vi "Main.vi"() -> ()   [LabVIEW 2017]
uses:
  CTL/REF Channel Select.ctl
  D:/test/ILSTS/LV_IL_Sample/DLL/STSProcess.dll
  DLL/STSProcess.dll
  CTL/Address Cluster.ctl
  D:/test/ILSTS/LV_IL_Sample/DLL/InstrumentDLL.dll
  DLL/InstrumentDLL.dll
  <vilib>/Utility/miscctls.llb/LVStringsAndValuesArrayTypeDef_DBL.ctl
panel:
  in  "ILSTS":refnum<k24>
  in  "btnzeroing":bool
  in  "btnreadref_data":bool
  in  "btnsaveRawdata":bool
  in  "btnsaveref_rawdata":bool
  in  "chkeach_ch":bool
  in  "btnmeas":bool
  in  "btnset":bool
  in  "Range1":bool
  in  "REF Channel Select":T1={"M1S0C1"=TRUE, "M1S0C2"=FALSE, "M1S0C3"=FALSE, "M1S0C4"=FALSE, "M1S1C1"=FALSE, "M1S1C2"=FALSE, "M1S1C3"=FALSE, "M1S1C4"=FALSE, "M1S2C1"=FALSE, "M1S2C2"=FALSE, "M1S2C3"=FALSE, "M1S2C4"=FALSE, "M1S3C1"=FALSE, "M1S3C2"=FALSE, "M1S3C3"=FALSE, "M1S3C4"=FALSE, "M1S4C1"=FALSE, "M1S4C2"=FALSE, "M1S4C3"=FALSE, "M1S4C4"=FALSE, "M2S0C1"=FALSE, "M2S0C2"=FALSE, "M2S0C3"=FALSE, "M2S0C4"=FALSE, "M2S1C1"=FALSE, "M2S1C2"=FALSE, "M2S1C3"=FALSE, "M2S1C4"=FALSE, "M2S2C1"=FALSE, "M2S2C2"=FALSE, "M2S2C3"=FALSE, "M2S2C4"=FALSE, "M2S3C1"=FALSE, "M2S3C2"=FALSE, "M2S3C3"=FALSE, "M2S3C4"=FALSE, "M2S4C1"=FALSE, "M2S4C2"=FALSE, "M2S4C3"=FALSE, "M2S4C4"=FALSE}
  in  "Range2":bool
  in  "Range3":bool
  in  "Range4":bool
  in  "Range5":bool
  in  "btnget_reference":bool
  in  "Address Cluster":T2={"SPU"=refnum, "MPM"=[], "Port_Count"=0.0, "MPM_Count"=0.0, "SPU_Resource"=[], "USB_Resource"=[], "MPM_Communicater"="", "MPM_Count"=0.0, "MPM_Address"=[], "MPM_Portnumber"=[], "SPU_DeviveID"="", "MPM_communcation_method"=[], "TSL_sweepstartwave"=0.0, "TSL_sweepstopwave"=0.0, "TSL_Address"="", "TSL_Communicater"="", "TSL"=refnum, "tsl_communcation_method"=3, "TSL_Portnumber"=0.0} {"tsl_communcation_method" items=["GPIB", "C232C", "TCPIP", "USB"]; "MPM_communcation_method" items=["GPIB", "C232C", "TCPIP", "USB"]}
  in  "Active Sensors":bool[](array[boolean])
  out "Meas_rang":i32[](array[numeric])
  out "Flag_213":bool
  out "Flag_215":bool
  out "Mergedata_struct":refnum<k24>[](array[refnum])
  out "Meas_monitor_struct":refnum<k24>[](array[refnum])
  out "Ref_monitordata_struct":refnum<k24>[](array[refnum])
  out "Refdata_struct":refnum<k24>[](array[refnum])
  out "Data_struct":refnum<k24>[](array[refnum])
  in  "txtpower":dbl caption="TSL Power(dBm)"
  in  "cmbspeed":u16(ring) caption="SweepSpeed(nm/sec)" items=["1"=1, "5"=5, "10"=10, "20"=20, "40"=40, "50"=50, "80"=80, "100"=100]
  in  "txtstepwave":dbl caption="WavelengthStep(nm)"
  in  "txtstopwave":dbl caption="StopWavelength(nm)"
  in  "txtstartwave":dbl caption="StartWavelength(nm)"
  # "Measurement ch"
  # "Measurement Range"
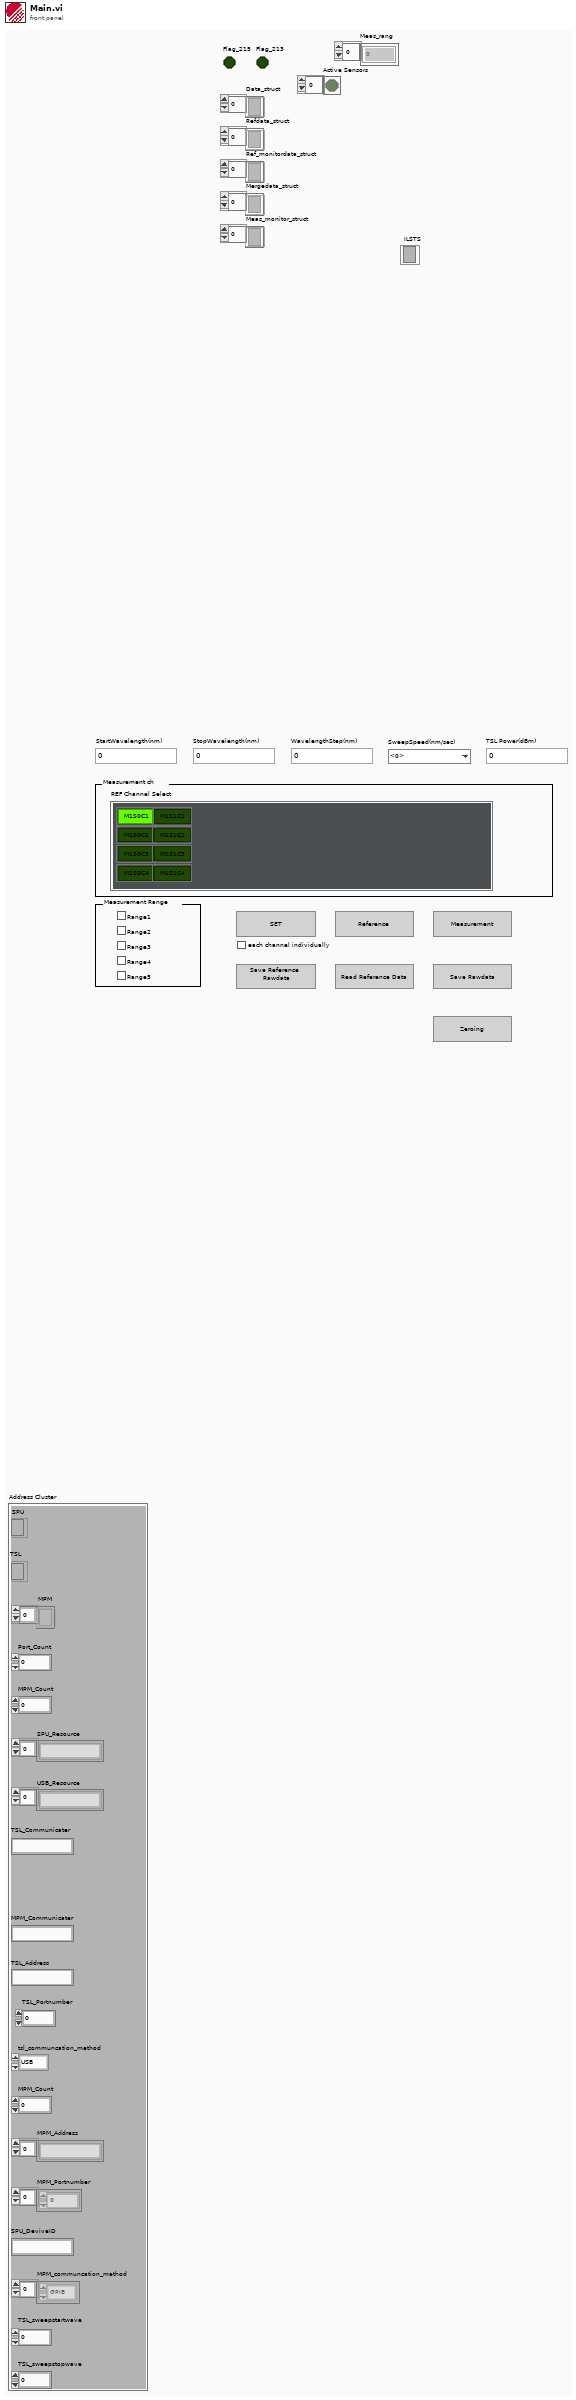
[diagram p1: front panel]
types:
  T1 = typedef "REF Channel Select.ctl" = cluster{"M1S0C1":bool, "M1S0C2":bool, "M1S0C3":bool, "M1S0C4":bool, "M1S1C1":bool, "M1S1C2":bool, "M1S1C3":bool, "M1S1C4":bool, "M1S2C1":bool, "M1S2C2":bool, "M1S2C3":bool, "M1S2C4":bool, "M1S3C1":bool, "M1S3C2":bool, "M1S3C3":bool, "M1S3C4":bool, "M1S4C1":bool, "M1S4C2":bool, "M1S4C3":bool, "M1S4C4":bool, "M2S0C1":bool, "M2S0C2":bool, "M2S0C3":bool, "M2S0C4":bool, "M2S1C1":bool, "M2S1C2":bool, "M2S1C3":bool, "M2S1C4":bool, "M2S2C1":bool, "M2S2C2":bool, "M2S2C3":bool, "M2S2C4":bool, "M2S3C1":bool, "M2S3C2":bool, "M2S3C3":bool, "M2S3C4":bool, "M2S4C1":bool, "M2S4C2":bool, "M2S4C3":bool, "M2S4C4":bool}
  T2 = typedef "Address Cluster.ctl" = cluster{"SPU":refnum<k24>, "MPM":refnum<k24>[], "Port_Count":dbl, "MPM_Count":dbl, "SPU_Resource":string[], "USB_Resource":string[], "MPM_Communicater":string, "MPM_Count":dbl, "MPM_Address":string[], "MPM_Portnumber":dbl[], "SPU_DeviveID":string, "MPM_communcation_method":i32[], "TSL_sweepstartwave":dbl, "TSL_sweepstopwave":dbl, "TSL_Address":string, "TSL_Communicater":string, "TSL":refnum<k24>, "tsl_communcation_method":i32, "TSL_Portnumber":dbl}
  T3 = enum8{"Enabled", "Disabled", "Disabled and Grayed Out"}
  T4 = typedef "LVStringsAndValuesArrayTypeDef_DBL.ctl" = cluster{"String":string, "Value":dbl}[]
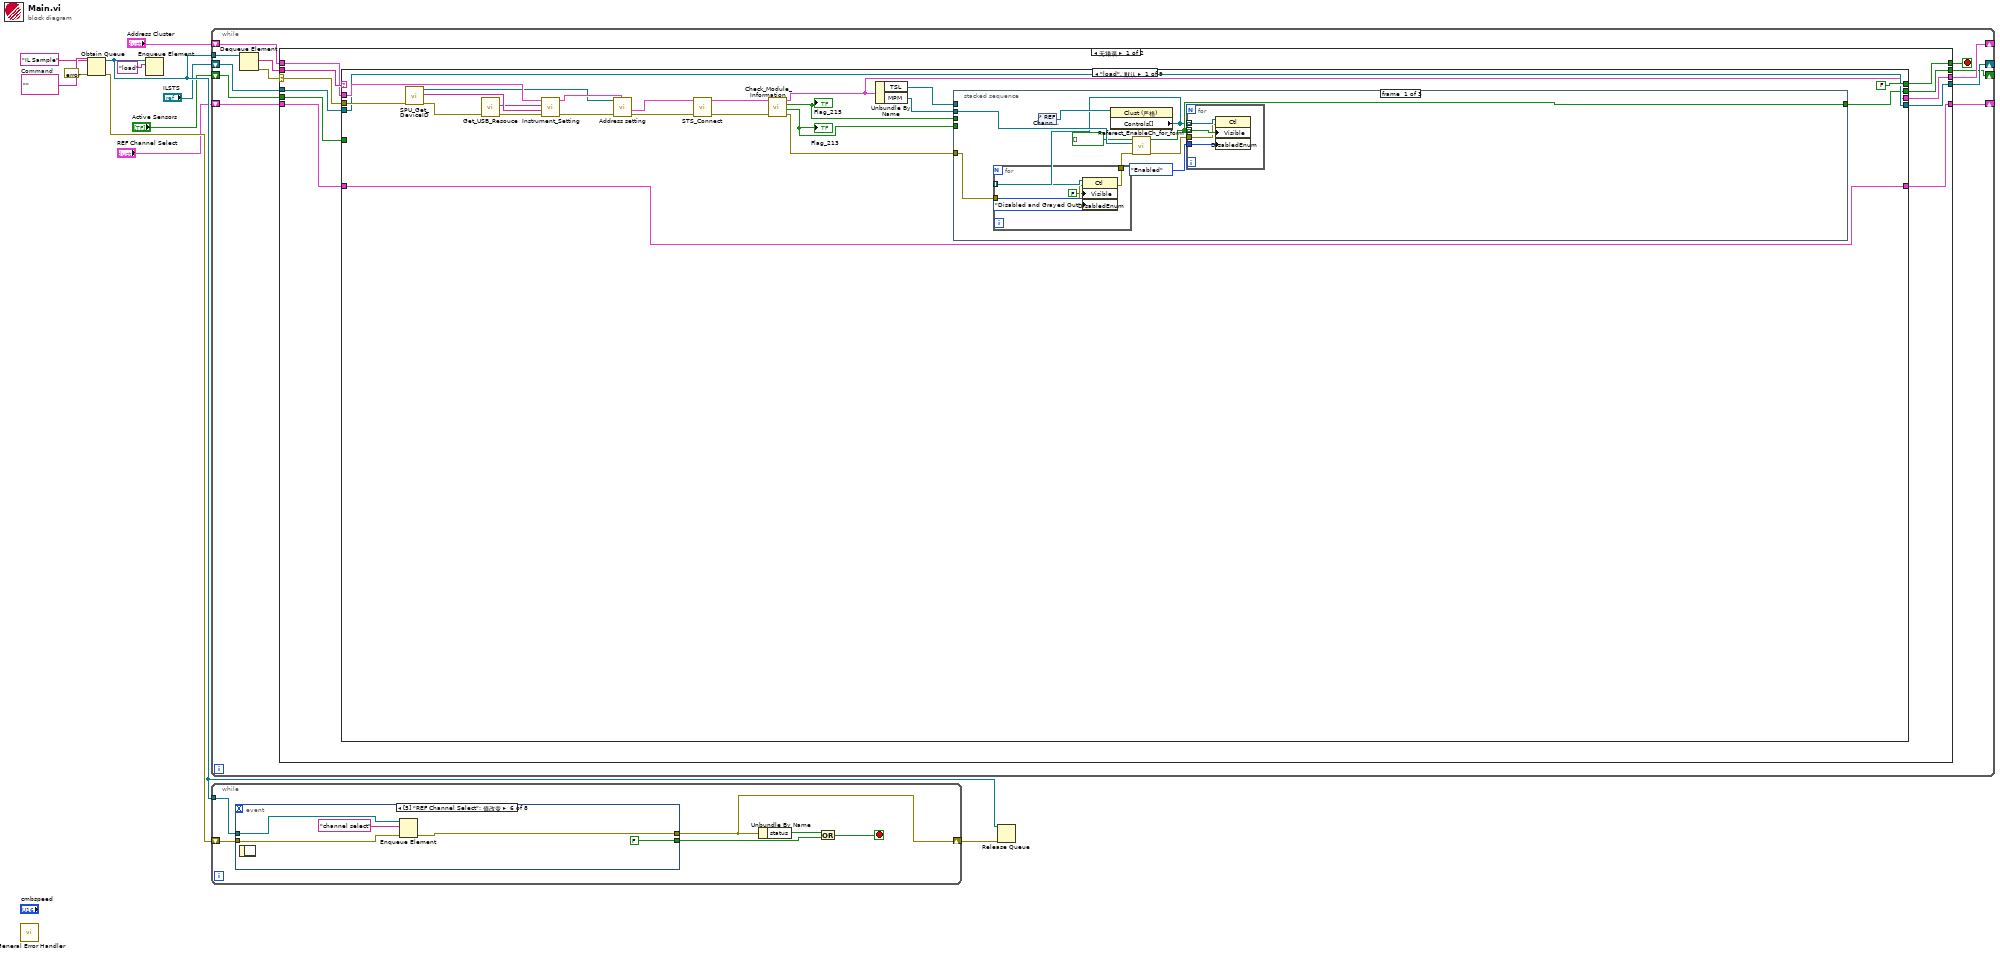
[diagram p0: block diagram]
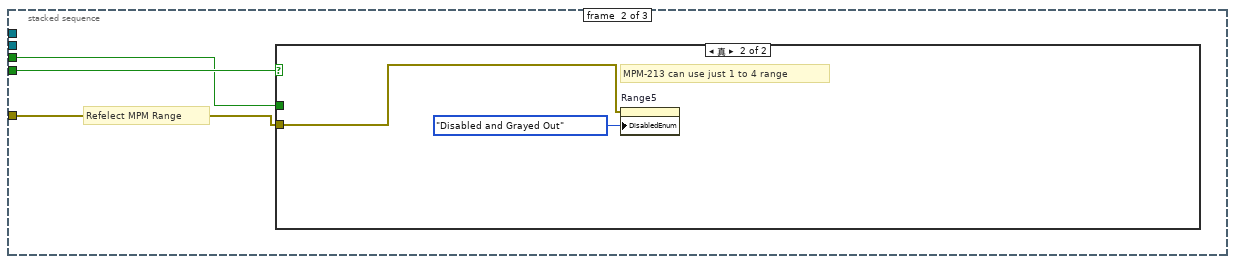
[diagram p2: hidden frame]
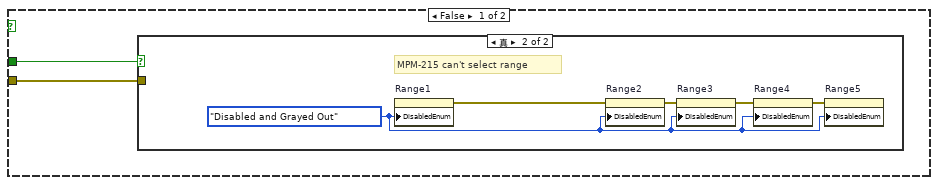
[diagram p3: hidden frame]
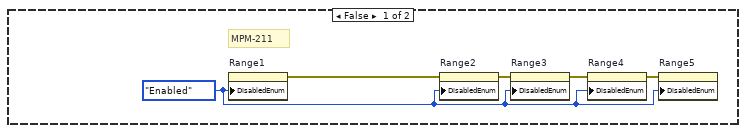
[diagram p4: hidden frame]
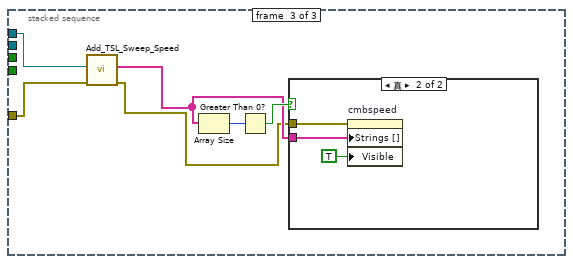
[diagram p5: hidden frame]
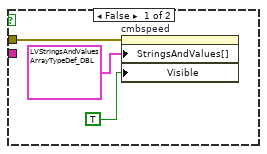
[diagram p6: hidden frame]
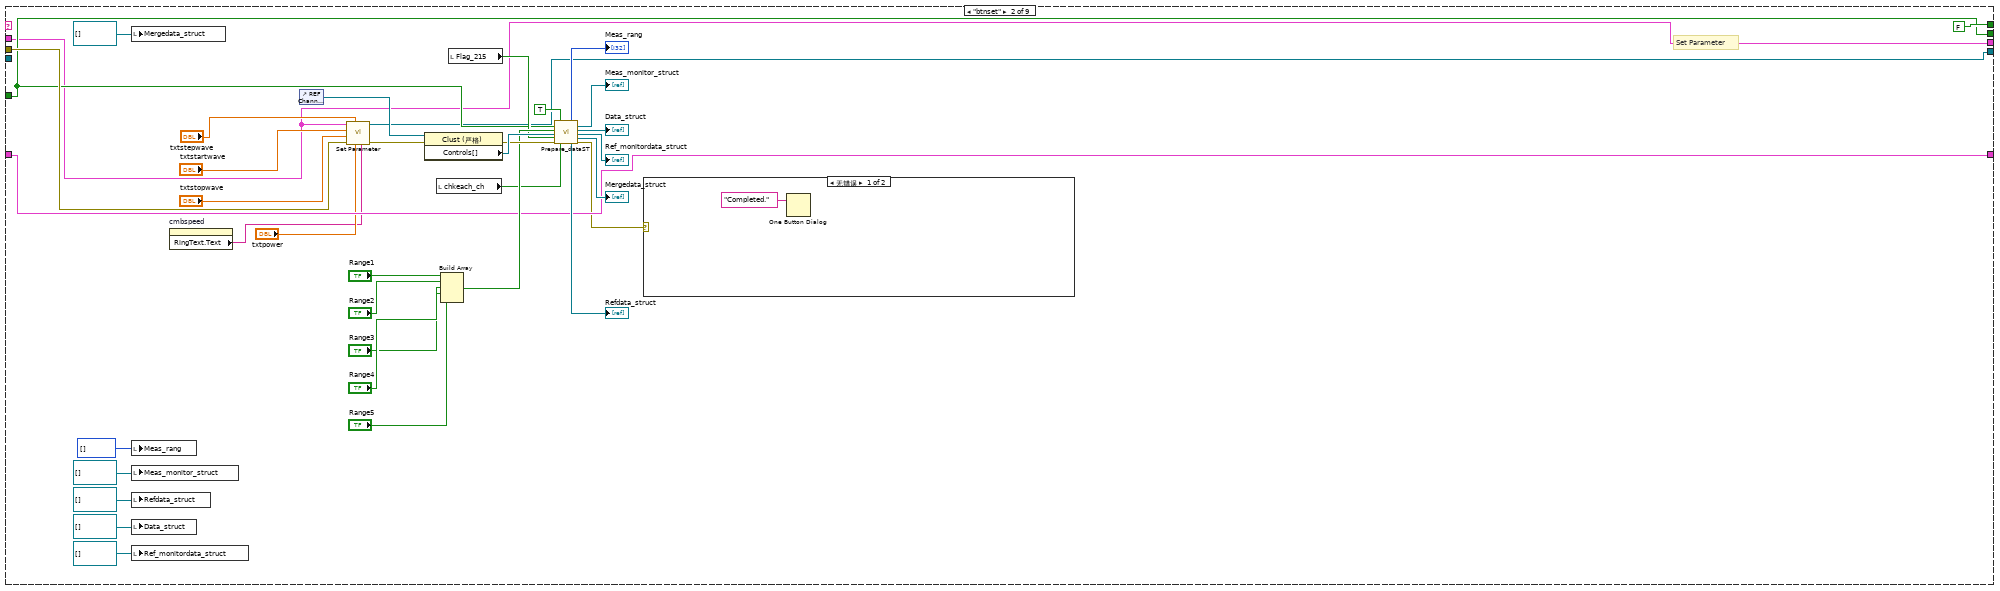
[diagram p7: hidden frame]
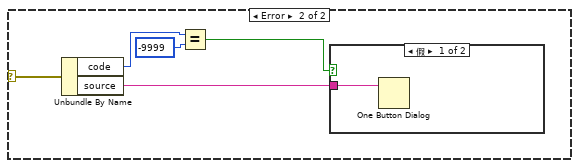
[diagram p8: hidden frame]
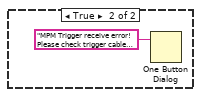
[diagram p9: hidden frame]
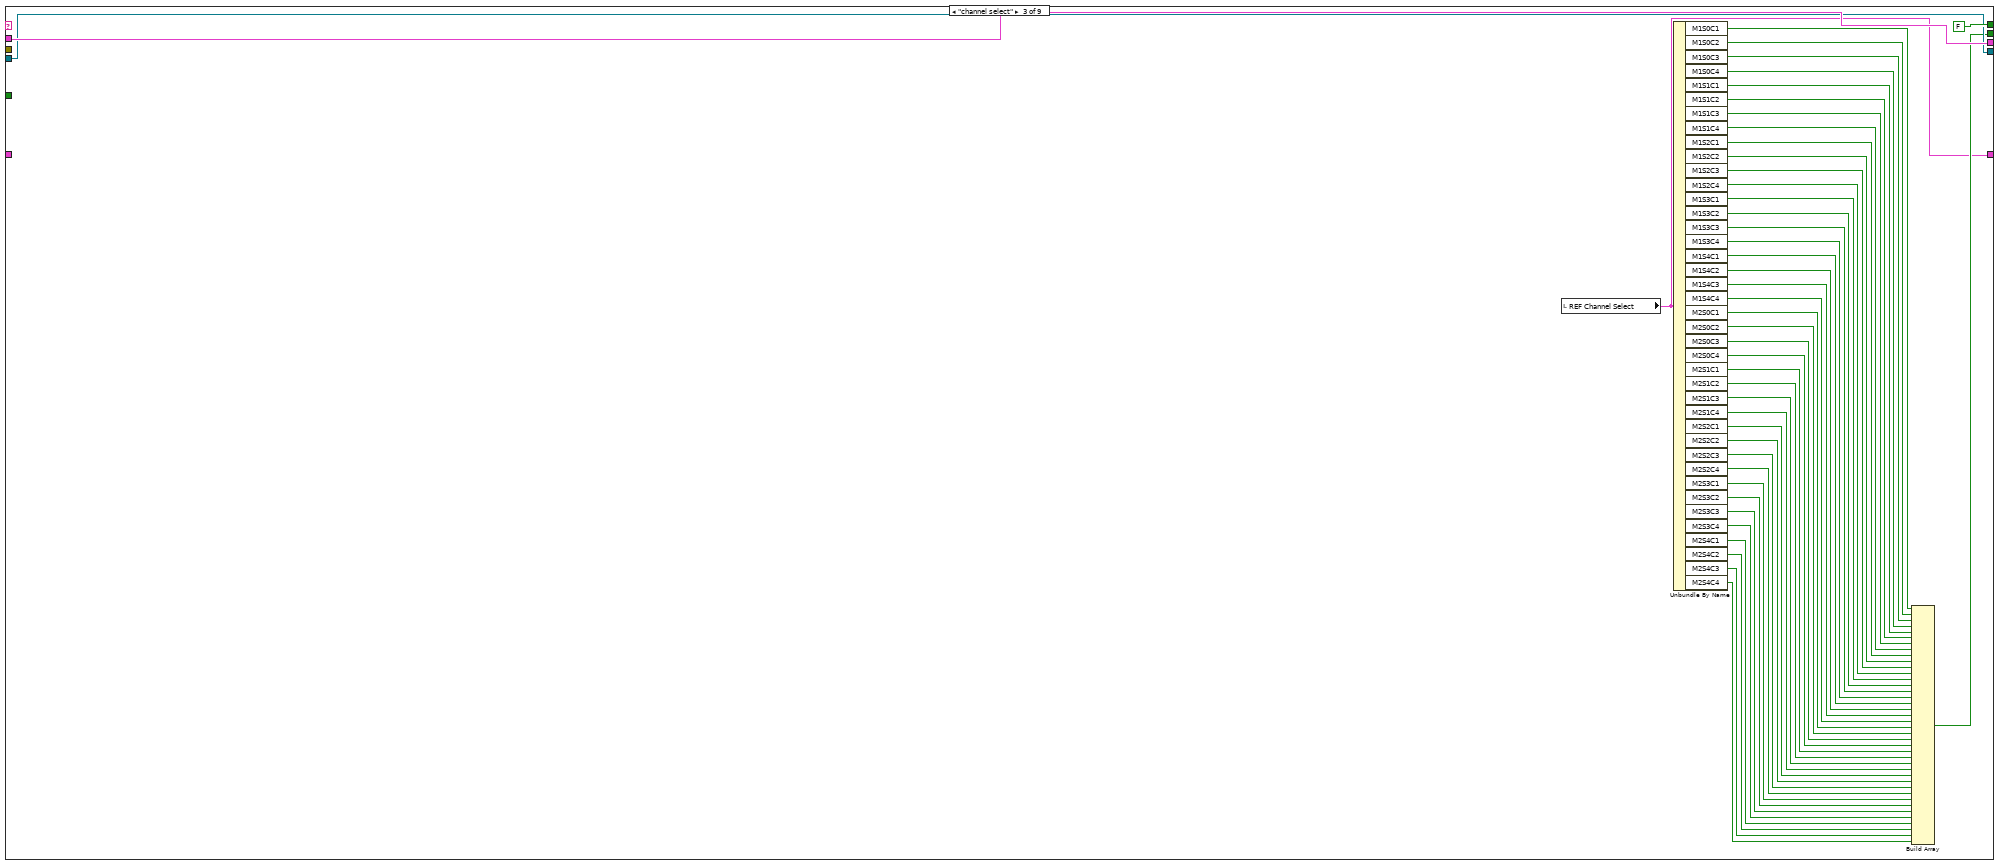
[diagram p10: hidden frame]
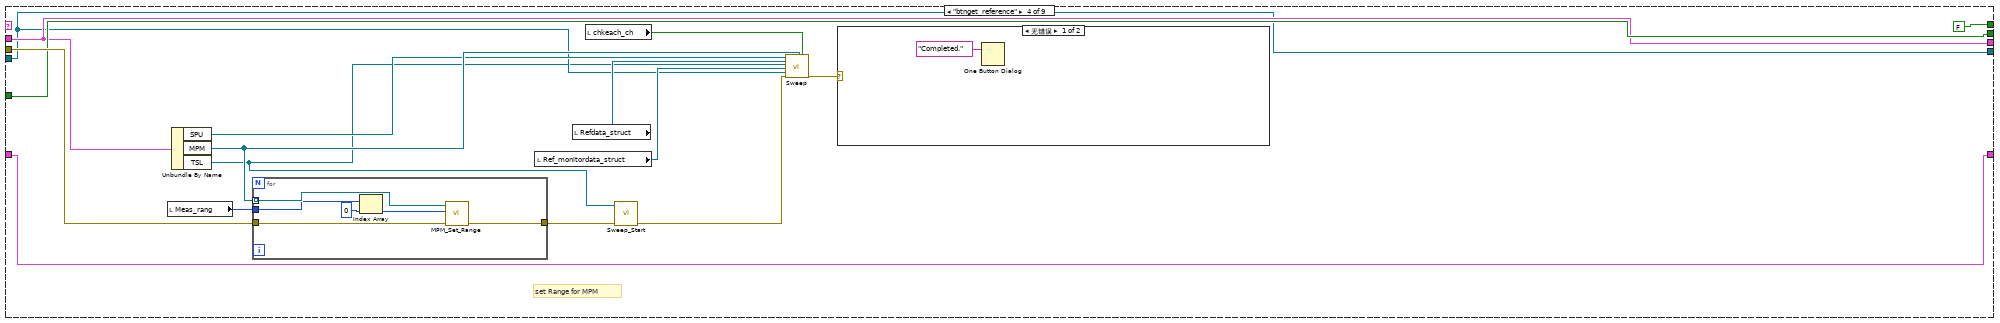
[diagram p11: hidden frame]
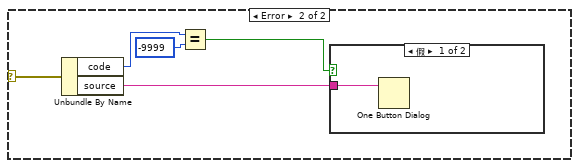
[diagram p12: hidden frame]
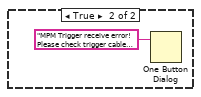
[diagram p13: hidden frame]
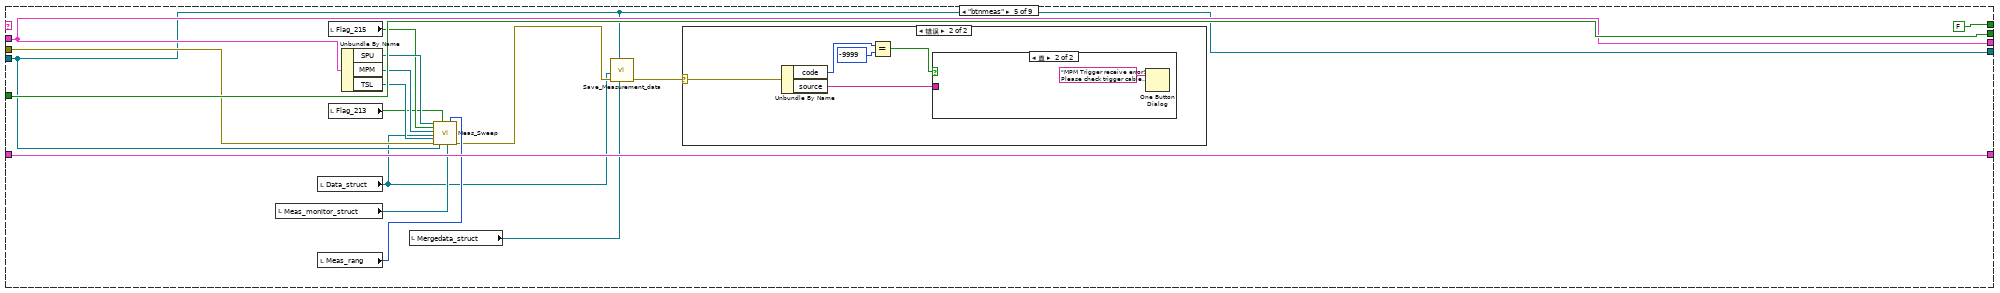
[diagram p14: hidden frame]
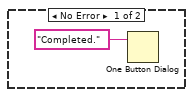
[diagram p15: hidden frame]
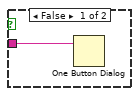
[diagram p16: hidden frame]
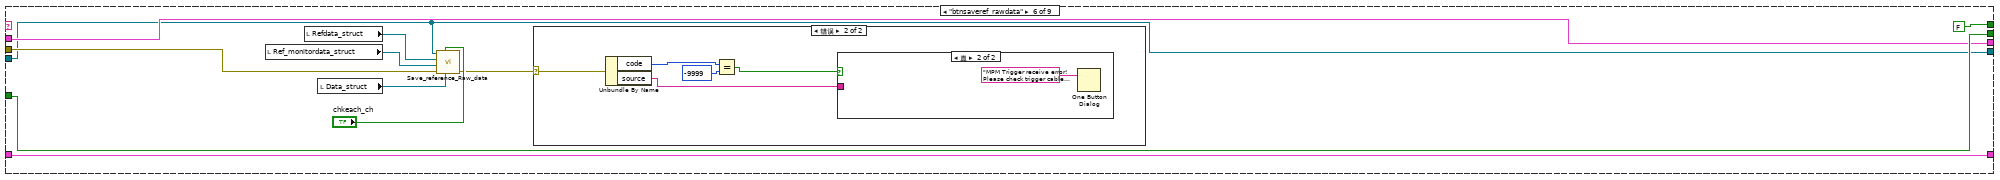
[diagram p17: hidden frame]
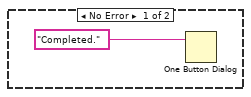
[diagram p18: hidden frame]
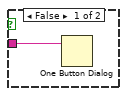
[diagram p19: hidden frame]
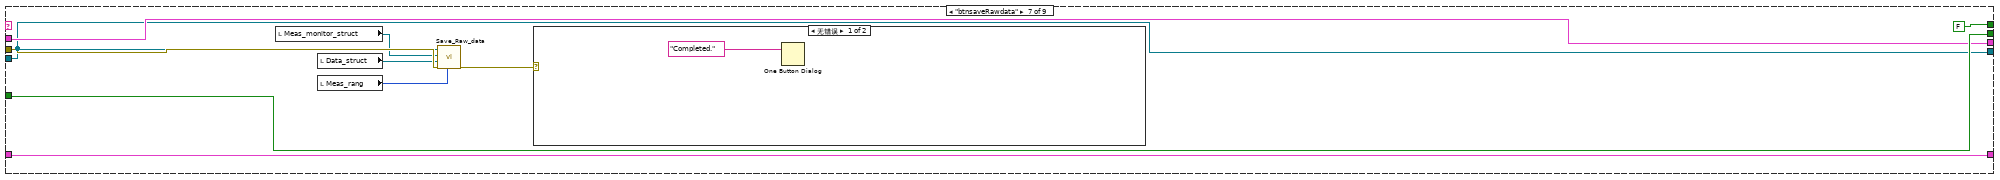
[diagram p20: hidden frame]
diagram:
  w11 = ""  # Command
  n1 = call <vilib>:"General Error Handler.vi"() -> ()  [unwired: 11 in, 5 out]
  n2 = Obtain Queue(name (unnamed)="IL Sample" ("名称（未命名）"), element data type=w11, error in (no error)=errorcluster {"status"=FALSE, "code"=0, "source"=""} ("错误输入（无错误）")) -> (queue out=w6:refnum<queue>, error out=w8:errorcluster)  [unwired: 2 in, 1 out]
  n3 = Enqueue Element(queue=w6, element="load" ("元素")) -> ()  [unwired: 2 in, 3 out]
  n4 = while {
    tunnel: w6 -> [w22]
    shift-right: [w18] -> _
    shift-left: "Address Cluster" -> [w19]
    shift-right: [w16] -> _
    shift-left: "ILSTS" -> [w17]
    shift-right: [w15] -> _
    shift-left: "Active Sensors" -> [w14]
    shift-right: [w12] -> _
    shift-left: "REF Channel Select" -> [w13]
    stop <- w20 stop-if-true
    n5 = Dequeue Element(queue=w22) -> (element=w21:string, error out=w23:errorcluster)  [unwired: 2 in, 2 out]
    n6 = case shown="无错误" w23 {
      selector: w23 -> [w31 _]
      tunnel: w21 -> [w34 _]
      tunnel: [w33 TRUE] -> w20
      tunnel: w19 -> [w32 w327]
      tunnel: [w26 w327] -> w18
      tunnel: w17 -> [w30 w325]
      tunnel: [w29 w325] -> w16
      tunnel: [w28 w326] -> w15
      tunnel: w14 -> [w27 w326]
      tunnel: w13 -> [w25 w324]
      tunnel: [w24 w324] -> w12
      frame No Error {
        n7 = case shown="\"load\", 默认" w34 {
          tunnel: [FALSE FALSE FALSE FALSE FALSE FALSE FALSE FALSE FALSE] -> w33
          tunnel: w32 -> [w57 w107 w193 w201 w240 w259 w277 w290 w313]
          tunnel: [w35 w107 w193 w201 w240 w259 w277 w290 w313] -> w26
          tunnel: w31 -> [w56 w121 _ w209 w238 w257 w275 w288 w307]
          tunnel: w30 -> [w43 _ w192 w196 w226 w253 w271 w291 w311]
          tunnel: [w43 w106 w192 w196 w226 w253 w271 w291 w311] -> w29
          tunnel: [w42 w120 w151 w202 w241 w260 w278 w294 w308] -> w28
          tunnel: w27 -> [_ w120 _ w202 w241 w260 w278 w294 w308]
          tunnel: w25 -> [w37 w119 _ w199 w237 w256 w274 w292 w314]
          tunnel: [w37 w119 w150 w199 w237 w256 w274 w292 w314] -> w24
          frame "load", Default {
            n8 = call "SPU_Get_DeviceID.vi"("错误输入（无错误）"=w56) -> ("error IO"=w53:errorcluster, "id"=w54:string[], "引用输出"=w48:refnum<k24>)  [unwired: 7 in]
            n9 = call "Get_USB_Resouce.vi"("error in (no error)"=w53) -> ("error out"=w47:errorcluster, "Get_USB_Resouce"=w52:string[])  [unwired: 8 in, 1 out]
            n10 = call "Instrument_Setting.vi"(8:w47, "id"=w54, "Get_USB_Resouce"=w52, "Address Cluster"=w57) -> ("错误输出"=w46:errorcluster, "Address Cluster out"=w51:T2)  [unwired: 6 in]
            n11 = call "Address setting.vi"("Address Cluster out输入"=w51, "错误输入（无错误）"=w46, "SPU in"=w48) -> ("error out"=w45:errorcluster, "Address Cluster out输出"=w50:T2)  [unwired: 7 in]
            n12 = call "STS_Connect.vi"("error in"=w45, "Address Cluster out输入"=w50) -> ("error out"=w44:errorcluster, "Address Cluster out"=w49:T2)  [unwired: 8 in]
            n13 = call "Check_Module_Information.vi"("Address Cluster"=w49, "错误输入（无错误）"=w44) -> ("Address Cluster out"=w35:T2, "Flag_215"=w40:bool, "Flag_213"=w41:bool, "error out"=w39:errorcluster)  [unwired: 5 in]
            "Flag_215" <- w40
            "Flag_213" <- w41
            n14 = Unbundle By Name(w35) -> ("TSL"=w38:refnum<k24>, "MPM"=w36:refnum<k24>[])
            n15 = stacked-sequence {
              tunnel: w36 -> [w66 _ _]
              tunnel: [w61 _ _] -> w42
              tunnel: w41 -> [_ w78 _]
              tunnel: w40 -> [_ w77 _]
              tunnel: w39 -> [w59 w76 w93]
              tunnel: w38 -> [_ _ w98]
              frame #0 {
                n16 = control-ref of="REF Channel Select"() -> (w64:refnum<vi>)
                n17 = property on="Property Node" class="Clust (严格)"(reference=w64) -> ("Controls[]"=w60:refnum<vi>[])  [unwired: 1 in, 2 out]
                n18 = for {
                  tunnel: w60 -> [w71] mode=indexing
                  tunnel: w59 -> [w70]
                  tunnel: [w69] -> w58
                  n19 = property on="Property Node" class="Ctl"(reference=w71, error in=w70, "Visible"=FALSE ("可见"), "DisabledEnum"=T3."Disabled and Grayed Out" ("禁用")) -> (error out=w69:errorcluster)  [unwired: 1 out]
                }
                n20 = call "Referect_EnableCh_for_form.vi"("错误输入（无错误）"=w58, "MPM"=w66, "数组输入"=bool[] []) -> ("error IO"=w62:errorcluster, "数组输出"=w61:bool[])  [unwired: 7 in]
                n21 = for {
                  tunnel: w60 -> [w75] mode=indexing
                  tunnel: w61 -> [w74] mode=indexing
                  tunnel: T3."Enabled" ("禁用") -> [w73]
                  tunnel: w62 -> [w72]
                  n22 = property on="Property Node" class="Ctl"(reference=w75, error in=w72, "Visible"=w74, "DisabledEnum"=w73) -> ()  [unwired: 2 out]
                }
              }
              frame #1 {
                # "Refelect MPM Range"
                n23 = case shown="真" w78 {
                  tunnel: w77 -> [w80 _]
                  tunnel: w76 -> [w79 w91]
                  frame False {
                    n24 = case shown="真" w80 {
                      tunnel: w79 -> [_ _]
                      frame False {
                        w81 = T3."Enabled" ("禁用")
                        # "MPM-211"
                        n25 = property on="Range1" class="Bool (严格)"("DisabledEnum"=w81) -> (error out=w85:errorcluster)  [unwired: 2 in, 1 out]
                        n26 = property on="Range2" class="Bool (严格)"(error in=w85, "DisabledEnum"=w81) -> (error out=w84:errorcluster)  [unwired: 1 in, 1 out]
                        n27 = property on="Range3" class="Bool (严格)"(error in=w84, "DisabledEnum"=w81) -> (error out=w83:errorcluster)  [unwired: 1 in, 1 out]
                        n28 = property on="Range4" class="Bool (严格)"(error in=w83, "DisabledEnum"=w81) -> (error out=w82:errorcluster)  [unwired: 1 in, 1 out]
                        n29 = property on="Range5" class="Bool (严格)"(error in=w82, "DisabledEnum"=w81) -> ()  [unwired: 1 in, 2 out]
                      }
                      frame True {
                        w86 = T3."Disabled and Grayed Out" ("禁用")
                        # "MPM-215 can't select range"
                        n30 = property on="Range1" class="Bool (严格)"("DisabledEnum"=w86) -> (error out=w90:errorcluster)  [unwired: 2 in, 1 out]
                        n31 = property on="Range2" class="Bool (严格)"(error in=w90, "DisabledEnum"=w86) -> (error out=w89:errorcluster)  [unwired: 1 in, 1 out]
                        n32 = property on="Range3" class="Bool (严格)"(error in=w89, "DisabledEnum"=w86) -> (error out=w88:errorcluster)  [unwired: 1 in, 1 out]
                        n33 = property on="Range4" class="Bool (严格)"(error in=w88, "DisabledEnum"=w86) -> (error out=w87:errorcluster)  [unwired: 1 in, 1 out]
                        n34 = property on="Range5" class="Bool (严格)"(error in=w87, "DisabledEnum"=w86) -> ()  [unwired: 1 in, 2 out]
                      }
                    }
                  }
                  frame True {
                    # "MPM-213 can use just 1 to 4 range"
                    n35 = property on="Range5" class="Bool (严格)"(error in=w91, "DisabledEnum"=T3."Disabled and Grayed Out" ("禁用")) -> ()  [unwired: 1 in, 2 out]
                  }
                }
              }
              frame #2 {
                n36 = call "Add_TSL_Sweep_Speed.vi"("TSL"=w98, "error in (no error)"=w93) -> ("数组输出"=w95:string[], "error out"=w94:errorcluster)  [unwired: 7 in]
                n37 = Array Size(array=w95) -> (size(s)=w97:i32)
                n38 = Greater Than 0?(x=w97) -> (x > 0?=w96:bool)
                n39 = case shown="真" w96 {
                  tunnel: w94 -> [w100 w103]
                  tunnel: w95 -> [_ w102]
                  frame False {
                    n40 = property on="cmbspeed" class="Ring (严格)"(error in=w100, "StringsAndValues[]"=T4 [{"String"="1", "Value"=1.0}, {"String"="5", "Value"=5.0}, {"String"="10", "Value"=10.0}, {"String"="20", "Value"=20.0}, {"String"="40", "Value"=40.0}, {"String"="50", "Value"=50.0}, {"String"="80", "Value"=80.0}, {"String"="100", "Value"=100.0}] ("Strings And Values []"), "Visible"=TRUE ("可见")) -> ()  [unwired: 1 in, 2 out]
                  }
                  frame True {
                    n41 = property on="cmbspeed" class="Ring (严格)"(error in=w103, "Strings []"=w102, "Visible"=TRUE ("可见")) -> ()  [unwired: 1 in, 2 out]
                  }
                }
              }
            }
          }
          frame "btnset" {
            # "Set Parameter"
            n42 = local write "Mergedata_struct"(refnum<k24>[] [] ("Mergedata_struct")) -> ()
            n43 = local write "Meas_rang"(i32[] [] ("Meas_rang")) -> ()
            n44 = local write "Meas_monitor_struct"(refnum<k24>[] [] ("Meas_monitor_struct")) -> ()
            n45 = local write "Refdata_struct"(refnum<k24>[] [] ("Refdata_struct")) -> ()
            n46 = local write "Data_struct"(refnum<k24>[] [] ("Data_struct")) -> ()
            n47 = local write "Ref_monitordata_struct"(refnum<k24>[] [] ("Ref_monitordata_struct")) -> ()
            n48 = property on="cmbspeed" class="Ring (严格)"() -> ("RingText.Text"=w109:string)  [unwired: 2 in, 2 out]
            n49 = control-ref of="REF Channel Select"() -> (w140:refnum<vi>)
            n50 = call "Set Parameter.vi"("RingText.Text"=w109, "txtpower"="txtpower", "txtstepwave"="txtstepwave", "error in"=w121, "txtstopwave"="txtstopwave", "txtstartwave"="txtstartwave", "Address Cluster"=w107) -> ("error out"=w108:errorcluster, "ILSTS"=w106:refnum<k24>)  [unwired: 3 in]
            n51 = property class="Clust (严格)"(reference=w140, error in=w108) -> (error out=w130:errorcluster, "Controls[]"=w131:refnum<vi>[])  [unwired: 1 out]
            n52 = local read "chkeach_ch"() -> (w128:bool)
            n53 = Build Array("Range1", "Range2", "Range3", "Range4", "Range5") -> (w129:bool[])
            n54 = local read "Flag_215"() -> (w127:bool)
            n55 = call "Prepare_dataST.vi"("Active Sensors"=w120, "ranges"=w129, "Controls[]"=w131, "Flag_215"=w127, "error in"=w130, "struct"=TRUE, "chkeach_ch"=w128) -> ("Meas_rang"=→"Meas_rang":i32[], "Refdata_struct"=→"Refdata_struct":refnum<k24>[], "Meas_monitor_struct"=→"Meas_monitor_struct":refnum<k24>[], "Data_struct"=→"Data_struct":refnum<k24>[], "Ref_monitordata_struct"=→"Ref_monitordata_struct":refnum<k24>[], "Mergedata_struct"=→"Mergedata_struct":refnum<k24>[], "error out"=w105:errorcluster)  [unwired: 6 in]
            n56 = case shown="无错误" w105 {
              selector: w105 -> [_ w147]
              frame No Error {
                n57 = One Button Dialog(message="Completed." ("消息")) -> ()  [unwired: 1 in, 1 out]
              }
              frame Error {
                n58 = Unbundle By Name(w147) -> ("code"=w146:i32, "source"=w143:string)
                n59 = Equal?(x=w146, y=-9999) -> (x = y?=w144:bool)
                n60 = case shown="假" w144 {
                  tunnel: w143 -> [w148 _]
                  frame False {
                    n61 = One Button Dialog(message=w148) -> ()  [unwired: 1 in, 1 out]
                  }
                  frame True {
                    n62 = One Button Dialog(message="MPM Trigger receive error! Please check trigger cable connection." ("消息")) -> ()  [unwired: 1 in, 1 out]
                  }
                }
              }
            }
          }
          frame "channel select" {
            n63 = local read "REF Channel Select"() -> (w150:T1)
            n64 = Unbundle By Name(w150) -> ("M1S0C1"=w191:bool, "M1S0C2"=w190:bool, "M1S0C3"=w189:bool, "M1S0C4"=w188:bool, "M1S1C1"=w187:bool, "M1S1C2"=w186:bool, "M1S1C3"=w185:bool, "M1S1C4"=w184:bool, "M1S2C1"=w183:bool, "M1S2C2"=w182:bool, "M1S2C3"=w181:bool, "M1S2C4"=w180:bool, "M1S3C1"=w179:bool, "M1S3C2"=w178:bool, "M1S3C3"=w177:bool, "M1S3C4"=w176:bool, "M1S4C1"=w175:bool, "M1S4C2"=w174:bool, "M1S4C3"=w173:bool, "M1S4C4"=w172:bool, "M2S0C1"=w171:bool, "M2S0C2"=w170:bool, "M2S0C3"=w169:bool, "M2S0C4"=w168:bool, "M2S1C1"=w167:bool, "M2S1C2"=w166:bool, "M2S1C3"=w165:bool, "M2S1C4"=w164:bool, "M2S2C1"=w163:bool, "M2S2C2"=w162:bool, "M2S2C3"=w161:bool, "M2S2C4"=w160:bool, "M2S3C1"=w159:bool, "M2S3C2"=w158:bool, "M2S3C3"=w157:bool, "M2S3C4"=w156:bool, "M2S4C1"=w155:bool, "M2S4C2"=w154:bool, "M2S4C3"=w153:bool, "M2S4C4"=w152:bool)
            n65 = Build Array(w191, w190, w189, w188, w187, w186, w185, w184, w183, w182, w181, w180, w179, w178, w177, w176, w175, w174, w173, w172, w171, w170, w169, w168, w167, w166, w165, w164, w163, w162, w161, w160, w159, w158, w157, w156, w155, w154, w153, w152) -> (w151:bool[])
          }
          frame "btnget_reference" {
            # "set Range for MPM"
            n66 = local read "Meas_rang"() -> (w210:i32[])
            n67 = Unbundle By Name(w201) -> ("SPU"=w206:refnum<k24>, "MPM"=w207:refnum<k24>[], "TSL"=w195:refnum<k24>)
            n68 = for {
              tunnel: w207 -> [w224] mode=indexing
              tunnel: w210 -> [w223]
              tunnel: w209 -> [w220]
              tunnel: [w219] -> w198
              n69 = Index Array(array=w223, index=0 ("索引")) -> (element=w221:i32)
              n70 = call "MPM_Set_Range.vi"("error in (no error)"=w220, "Range All"=w221, ".NET Reference in"=w224) -> ("error out"=w219:errorcluster)  [unwired: 7 in, 1 out]
            }
            n71 = local read "Ref_monitordata_struct"() -> (w203:refnum<k24>[])
            n72 = local read "Refdata_struct"() -> (w204:refnum<k24>[])
            n73 = local read "chkeach_ch"() -> (w208:bool)
            n74 = call "Sweep_Start.vi"("error in (no error)"=w198, ".NET Reference in"=w195) -> ("error out"=w197:errorcluster)  [unwired: 8 in, 1 out]
            n75 = call "Sweep.vi"("SPU"=w206, "Refdata_struct"=w204, "TSL"=w195, "Ref_monitordata_struct"=w203, "ILSTS"=w196, "错误输入（无错误）"=w197, "MPM"=w207, "chkeach_ch"=w208) -> ("错误输出"=w205:errorcluster)  [unwired: 11 in]
            n76 = case shown="无错误" w205 {
              selector: w205 -> [_ w216]
              frame No Error {
                n77 = One Button Dialog(message="Completed." ("消息")) -> ()  [unwired: 1 in, 1 out]
              }
              frame Error {
                n78 = Unbundle By Name(w216) -> ("code"=w215:i32, "source"=w212:string)
                n79 = Equal?(x=w215, y=-9999) -> (x = y?=w213:bool)
                n80 = case shown="假" w213 {
                  tunnel: w212 -> [w217 _]
                  frame False {
                    n81 = One Button Dialog(message=w217) -> ()  [unwired: 1 in, 1 out]
                  }
                  frame True {
                    n82 = One Button Dialog(message="MPM Trigger receive error! Please check trigger cable connection." ("消息")) -> ()  [unwired: 1 in, 1 out]
                  }
                }
              }
            }
          }
          frame "btnmeas" {
            n83 = local read "Meas_monitor_struct"() -> (w233:refnum<k24>[])
            n84 = local read "Data_struct"() -> (w225:refnum<k24>[])
            n85 = local read "Meas_rang"() -> (w235:i32[])
            n86 = local read "Flag_215"() -> (w231:bool)
            n87 = local read "Flag_213"() -> (w230:bool)
            n88 = Unbundle By Name(w240) -> ("SPU"=w234:refnum<k24>, "MPM"=w232:refnum<k24>[], "TSL"=w236:refnum<k24>)
            n89 = local read "Mergedata_struct"() -> (w227:refnum<k24>[])
            n90 = call "Meas_Sweep.vi"("SPU"=w234, "Flag_215"=w231, "MPM"=w232, "Data_struct"=w225, "TSL"=w236, "错误输入（无错误）"=w238, "ILSTS"=w226, "Flag_213"=w230, "Meas_monitor_struct"=w233, "Meas_rang"=w235) -> ("错误输出"=w229:errorcluster)  [unwired: 9 in]
            n91 = call "Save_Measurement_data.vi"("Mergedata_struct"=w227, "ILSTS"=w226, "错误输入（无错误）"=w229, "Data_struct"=w225) -> ("错误输出"=w228:errorcluster)  [unwired: 7 in]
            n92 = case shown="错误" w228 {
              selector: w228 -> [_ w247]
              frame No Error {
                n93 = One Button Dialog(message="Completed." ("消息")) -> ()  [unwired: 1 in, 1 out]
              }
              frame Error {
                n94 = Unbundle By Name(w247) -> ("code"=w246:i32, "source"=w243:string)
                n95 = Equal?(x=w246, y=-9999) -> (x = y?=w244:bool)
                n96 = case shown="真" w244 {
                  tunnel: w243 -> [w248 _]
                  frame False {
                    n97 = One Button Dialog(message=w248) -> ()  [unwired: 1 in, 1 out]
                  }
                  frame True {
                    n98 = One Button Dialog(message="MPM Trigger receive error! Please check trigger cable connection." ("消息")) -> ()  [unwired: 1 in, 1 out]
                  }
                }
              }
            }
          }
          frame "btnsaveref_rawdata" {
            n99 = local read "Ref_monitordata_struct"() -> (w251:refnum<k24>[])
            n100 = local read "Refdata_struct"() -> (w252:refnum<k24>[])
            n101 = local read "Data_struct"() -> (w254:refnum<k24>[])
            n102 = call "Save_reference_Raw_data.vi"("Data_struct"=w254, "chkeach_ch"="chkeach_ch", "错误输入（无错误）"=w257, "Ref_monitordata_struct"=w251, "Refdata_struct"=w252, "ILSTS"=w253) -> ("错误输出"=w250:errorcluster)  [unwired: 5 in]
            n103 = case shown="错误" w250 {
              selector: w250 -> [_ w266]
              frame No Error {
                n104 = One Button Dialog(message="Completed." ("消息")) -> ()  [unwired: 1 in, 1 out]
              }
              frame Error {
                n105 = Unbundle By Name(w266) -> ("code"=w265:i32, "source"=w262:string)
                n106 = Equal?(x=w265, y=-9999) -> (x = y?=w263:bool)
                n107 = case shown="真" w263 {
                  tunnel: w262 -> [w267 _]
                  frame False {
                    n108 = One Button Dialog(message=w267) -> ()  [unwired: 1 in, 1 out]
                  }
                  frame True {
                    n109 = One Button Dialog(message="MPM Trigger receive error! Please check trigger cable connection." ("消息")) -> ()  [unwired: 1 in, 1 out]
                  }
                }
              }
            }
          }
          frame "btnsaveRawdata" {
            n110 = local read "Meas_monitor_struct"() -> (w269:refnum<k24>[])
            n111 = local read "Data_struct"() -> (w270:refnum<k24>[])
            n112 = local read "Meas_rang"() -> (w273:i32[])
            n113 = call "Save_Raw_data.vi"("Meas_rang"=w273, "错误输入（无错误）"=w275, "Data_struct"=w270, "Meas_monitor_struct"=w269, "ILSTS"=w271) -> ("错误输出"=w272:errorcluster)  [unwired: 6 in]
            n114 = case shown="无错误" w272 {
              selector: w272 -> [_ w284]
              frame No Error {
                n115 = One Button Dialog(message="Completed." ("消息")) -> ()  [unwired: 1 in, 1 out]
              }
              frame Error {
                n116 = Unbundle By Name(w284) -> ("code"=w283:i32, "source"=w280:string)
                n117 = Equal?(x=w283, y=-9999) -> (x = y?=w281:bool)
                n118 = case shown="真" w281 {
                  tunnel: w280 -> [w285 _]
                  frame False {
                    n119 = One Button Dialog(message=w285) -> ()  [unwired: 1 in, 1 out]
                  }
                  frame True {
                    n120 = One Button Dialog(message="MPM Trigger receive error! Please check trigger cable connection." ("消息")) -> ()  [unwired: 1 in, 1 out]
                  }
                }
              }
            }
          }
          frame "btnzeroing" {
            n121 = Unbundle By Name(w290) -> ("MPM"=w289:refnum<k24>[])
            n122 = for {
              tunnel: w289 -> [w297] mode=indexing
              tunnel: w288 -> [w296]
              tunnel: [w295] -> w287
              n123 = call "MPM_Zeroing.vi"("error in (no error)"=w296, ".NET Reference in"=w297) -> ("error out"=w295:errorcluster)  [unwired: 8 in, 1 out]
            }
            n124 = case shown="错误" w287 {
              selector: w287 -> [_ w303]
              frame No Error {
                n125 = One Button Dialog(message="Completed." ("消息")) -> ()  [unwired: 1 in, 1 out]
              }
              frame Error {
                n126 = Unbundle By Name(w303) -> ("code"=w302:i32, "source"=w299:string)
                n127 = Equal?(x=w302, y=-9999) -> (x = y?=w300:bool)
                n128 = case shown="假" w300 {
                  tunnel: w299 -> [w304 _]
                  frame False {
                    n129 = One Button Dialog(message=w304) -> ()  [unwired: 1 in, 1 out]
                  }
                  frame True {
                    n130 = One Button Dialog(message="MPM Trigger receive error! Please check trigger cable connection." ("消息")) -> ()  [unwired: 1 in, 1 out]
                  }
                }
              }
            }
          }
          frame "btnreadref_data" {
            n131 = Unbundle By Name(w313) -> ("TSL"=w312:refnum<k24>)
            n132 = local read "chkeach_ch"() -> (w310:bool)
            n133 = local read "Data_struct"() -> (w309:refnum<k24>[])
            n134 = call "Reference_Data_Read.vi"("Active Sensors"=w308, "chkeach_ch"=w310, "error in"=w307, "ILSTS"=w311, "Data_struct"=w309, "TSL"=w312) -> ("error IO"=w306:errorcluster)  [unwired: 5 in]
            n135 = case shown="错误" w306 {
              selector: w306 -> [_ w321]
              frame No Error {
                n136 = One Button Dialog(message="Completed." ("消息")) -> ()  [unwired: 1 in, 1 out]
              }
              frame Error {
                n137 = Unbundle By Name(w321) -> ("code"=w320:i32, "source"=w317:string)
                n138 = Equal?(x=w320, y=-9999) -> (x = y?=w318:bool)
                n139 = case shown="假" w318 {
                  tunnel: w317 -> [w322 _]
                  frame False {
                    n140 = One Button Dialog(message=w322) -> ()  [unwired: 1 in, 1 out]
                  }
                  frame True {
                    n141 = One Button Dialog(message="MPM Trigger receive error! Please check trigger cable connection." ("消息")) -> ()  [unwired: 1 in, 1 out]
                  }
                }
              }
            }
          }
        }
      }
      frame Error {
      }
    }
  }
  n142 = while {
    tunnel: w6 -> [w333]
    shift-right: [w329] -> w7
    shift-left: w8 -> [w334]
    stop <- w331 stop-if-true
    n143 = event shown="[5] \"REF Channel Select\": 值改变" {
      selector: _ -> [_ _ _ _ _ _ _ _]
      dyn-events: _ -> [_ _ _ _ _ _ _ _]
      timeout: _ -> [_ _ _ _ _ _ _ _]
      tunnel: w334 -> [w337 w347 w352 w357 w362 w365 w370 w375]
      tunnel: w333 -> [w338 w346 w351 w356 w361 w363 w368 w373]
      tunnel: [w342 w345 w350 w355 w360 w364 w369 w374] -> w329
      tunnel: [FALSE FALSE FALSE FALSE FALSE FALSE FALSE FALSE] -> w330
      event "btnset": Value Change {
        n144 = event-data() -> ()  [unwired: 1 in, 1 out]
        n145 = Enqueue Element(queue=w338, element="channel select" ("元素"), error in (no error)=w337) -> (queue out=w335:refnum<queue>, error out=w336:errorcluster)  [unwired: 1 in, 1 out]
        n146 = Enqueue Element(queue=w335, element="btnset" ("元素"), error in (no error)=w336) -> (error out=w342:errorcluster)  [unwired: 1 in, 2 out]
      }
      event "btnget_reference": Value Change {
        n147 = event-data() -> ()  [unwired: 1 in, 1 out]
        n148 = Enqueue Element(queue=w346, element="btnget_reference" ("元素"), error in (no error)=w347) -> (error out=w345:errorcluster)  [unwired: 1 in, 2 out]
      }
      event "btnmeas": Value Change {
        n149 = event-data() -> ()  [unwired: 1 in, 1 out]
        n150 = Enqueue Element(queue=w351, element="btnmeas" ("元素"), error in (no error)=w352) -> (error out=w350:errorcluster)  [unwired: 1 in, 2 out]
      }
      event "btnzeroing": Value Change {
        n151 = event-data() -> ()  [unwired: 1 in, 1 out]
        n152 = Enqueue Element(queue=w356, element="btnzeroing" ("元素"), error in (no error)=w357) -> (error out=w355:errorcluster)  [unwired: 1 in, 2 out]
      }
      event "btnsaveref_rawdata": Value Change {
        n153 = event-data() -> ()  [unwired: 1 in, 1 out]
        n154 = Enqueue Element(queue=w361, element="btnsaveref_rawdata" ("元素"), error in (no error)=w362) -> (error out=w360:errorcluster)  [unwired: 1 in, 2 out]
      }
      event Value Change {
        n155 = event-data() -> ()  [unwired: 1 in, 1 out]
        n156 = Enqueue Element(queue=w363, element="channel select" ("元素"), error in (no error)=w365) -> (error out=w364:errorcluster)  [unwired: 1 in, 2 out]
      }
      event "btnreadref_data": Value Change {
        n157 = event-data() -> ()  [unwired: 1 in, 1 out]
        n158 = Enqueue Element(queue=w368, element="btnreadref_data" ("元素"), error in (no error)=w370) -> (error out=w369:errorcluster)  [unwired: 1 in, 2 out]
      }
      event "btnsaveRawdata": Value Change {
        n159 = event-data() -> ()  [unwired: 1 in, 1 out]
        n160 = Enqueue Element(queue=w373, element="btnsaveRawdata" ("元素"), error in (no error)=w375) -> (error out=w374:errorcluster)  [unwired: 1 in, 2 out]
      }
    }
    n161 = Unbundle By Name(w329) -> ("status"=w332:bool)
    n162 = Or(x=w332, y=w330) -> (x .or. y?=w331:bool)
  }
  n163 = Release Queue(queue=w6, error in (no error)=w7) -> ()  [unwired: 1 in, 3 out]
